vi "Object Tracking.vi"() -> ()   [LabVIEW 2019]
doc: "This example demonstrates the Traditional MeanShift algorithm to track an object in the image."
panel:
  in  "Stop":bool
  in  "Delay (s.)":dbl(slide) scale=0.0..2.0
  out "Image":T1(plugin-control)
  # "Overview: Demonstrate the Traditional MeanShift algorithm to track an object in the image.\nRequirements: LabVIEW Full Development System and Vision Development Module.\nInstructions: Run the VI."
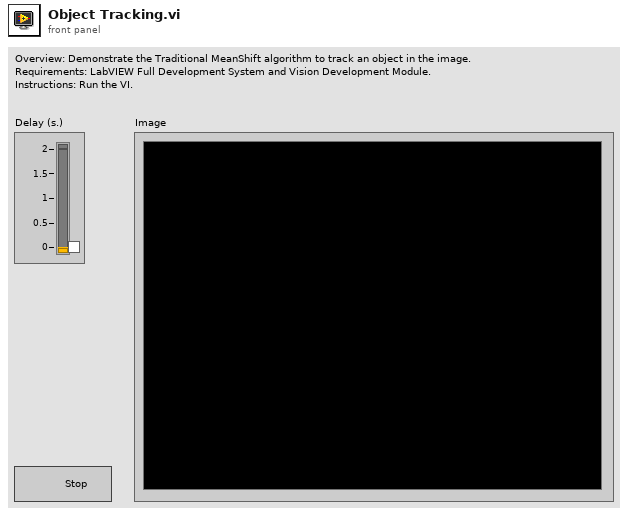
[diagram p1: front panel]
types:
  T1 = typedef "IMAQ Image.ctl" = refnum<image>
  T2 = cluster{"Number of Histogram Bins":i32, "Blending Parameter (%)":dbl, "Maximum Iterations":i32}
  T3 = typedef "Image Type" = u32
  T4 = typedef "IMAQ Object Tracking Session.ctl" = refnum<k20>
  T5 = typedef "IMAQ AVI2 Refnum.ctl" = refnum<k20>
  T6 = typedef "IMAQ Rectangle" = cluster{"Left":i32, "Top":i32, "Right":i32, "Bottom":i32, "Rotation":dbl}
  T7 = typedef "ROI Descriptor" = cluster{"Global Rectangle":i32[], "Contours":cluster{"ID":enum32{"External", "Internal"}, "Type":u32, "Coordinates":i32[]}[]}
  T8 = cluster{"Label":string, "Score":i32, "Angle":dbl, "Location":cluster{"X":dbl, "Y":dbl}, "Bounding Box":cluster{"X":dbl, "Y":dbl}[], "Object Found?":bool}[]
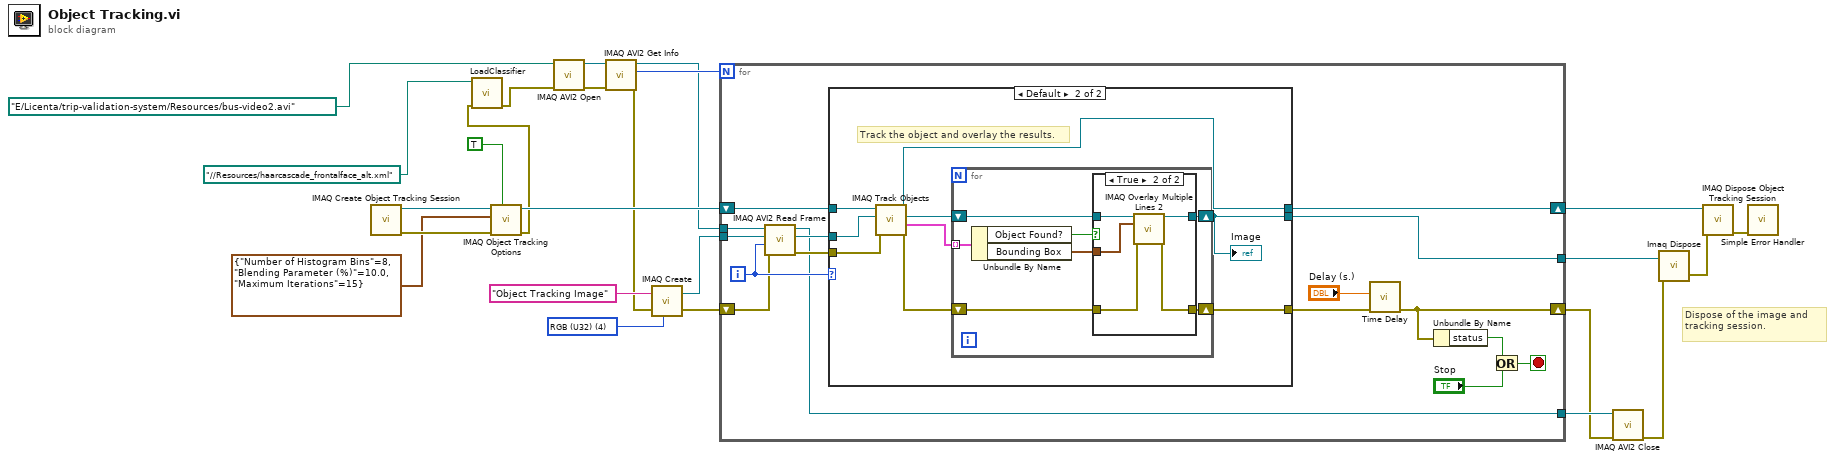
[diagram p0: block diagram]
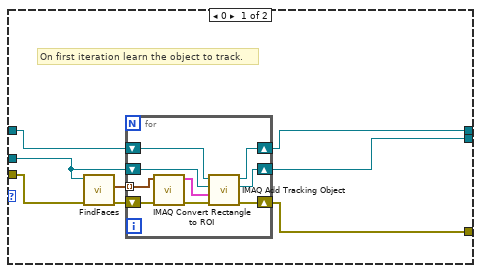
[diagram p2: hidden frame]
diagram:
  w12 = T3 4 items=["Grayscale (U8)", "Grayscale (I16)", "Grayscale (SGL)", "Complex (CSG)", "RGB (U32)", "HSL (U32)", "RGB (U64)", "Grayscale (U16)"] ("Image Type")
  # "Dispose of the image and tracking session."
  n1 = call "IMAQ Create Object Tracking Session"() -> ("error out"=w18:errorcluster, "Object Tracking Session"=w21:T4)  [unwired: 1 in, 9 out]
  n2 = call-poly "IMAQ Object Tracking Options"("Get/Set (Get)"=TRUE, "error in (no error)"=w18, "Mean Shift Options in"=T2 {"Number of Histogram Bins"=8, "Blending Parameter (%)"=10.0, "Maximum Iterations"=15}, "Object Tracking Session In"=w21) -> ("error out"=w4:errorcluster, "Object Tracking Session Out"=w20:T4)  [unwired: 5 in, 1 out]
  n3 = call "LoadClassifier.vi"("error in (no error)"=w4, "faceCascadePath"=path "../../Resources/haarcascade_frontalface_alt.xml" ("Face Cascade Path")) -> ("error out"=w3:errorcluster)  [unwired: 9 in]
  n4 = call "IMAQ AVI2 Open"("error in (no error)"=w3, "AVI File Path"=path "E:/Licenta/trip-validation-system/Resources/bus-video2.avi") -> ("error out"=w16:errorcluster, "AVI Refnum"=w17:T5)  [unwired: 8 in]
  n5 = call "IMAQ AVI2 Get Info"("error in (no error)"=w16, "AVI Refnum"=w17) -> ("error out"=w13:errorcluster, "Number of Frames"=w15:u32, "AVI Refnum (duplicate)"=w11:T5)  [unwired: 5 in, 2 out]
  n6 = call "IMAQ Create"("Image Name"="Object Tracking Image", "Image Type"=w12, "error in (no error)"=w13) -> ("New Image"=w10:T1, "error out"=w9:errorcluster)  [unwired: 2 in]
  n7 = for {
    N: w15 -> [_]
    tunnel: [w40] -> w25
    shift-right: [w38] -> w24
    shift-left: w20 -> [w39]
    tunnel: w11 -> [w35]
    tunnel: w10 -> [w34]
    shift-right: [w27] -> w7
    shift-left: w9 -> [w28]
    tunnel: [w26] -> w8
    i -> [w31]
    stop <- w29 stop-if-true
    n8 = call "IMAQ AVI2 Read Frame"("error in (no error)"=w28, "Frame Number"=w31, "Image"=w34, "AVI Refnum"=w35) -> ("error out"=w32:errorcluster, "Image Out"=w33:T1, "AVI Refnum (duplicate)"=w26:T5)  [unwired: 5 in]
    n9 = case shown="Default" w31 {
      tunnel: [w46 w67] -> w38
      tunnel: [w48 w65] -> w40
      tunnel: [w47 w62] -> w36
      tunnel: w39 -> [w49 w64]
      tunnel: w33 -> [w45 w61]
      tunnel: w32 -> [w44 w60]
      frame 0 {
        # "On first iteration learn the object to track."
        n10 = call "FindFaces.vi"("error in"=w44, "Image In"=w45) -> ("error out"=w43:errorcluster, "Faces"=w42:T6[])  [unwired: 7 in, 1 out]
        n11 = for {
          shift-right: [w55] -> w46
          shift-left: w49 -> [w58]
          shift-right: [w57] -> w48
          shift-left: w45 -> [w52]
          shift-right: [w56] -> w47
          shift-left: w43 -> [w51]
          tunnel: w42 -> [w50] mode=indexing
          n12 = call "IMAQ Convert Rectangle to ROI"("error in (no error)"=w51, "Rectangle"=w50) -> ("error out"=w54:errorcluster, "ROI Descriptor"=w53:T7)  [unwired: 7 in]
          n13 = call "IMAQ Add Tracking Object"("error in (no error)"=w54, "ROI Descriptor"=w53, "Image"=w52, "Object Tracking Session In"=w58) -> ("error out"=w56:errorcluster, "Image (duplicate)"=w57:T1, "Object Tracking Session Out"=w55:T4)  [unwired: 1 in, 4 out]
        }
      }
      frame Default {
        # "Track the object and overlay the results."
        n14 = call "IMAQ Track Objects"("error in (no error)"=w60, "Image"=w61, "Object Tracking Session In"=w64) -> ("error out"=w63:errorcluster, "Objects (pixel)"=w59:T8, "Image (duplicate)"=w66:T1, "Object Tracking Session Out"=w67:T4)  [unwired: 1 in, 4 out]
        n15 = for {
          shift-right: [w73] -> w65
          shift-left: w66 -> [w74]
          shift-right: [w70] -> w62
          shift-left: w63 -> [w71]
          tunnel: w59 -> [w68] mode=indexing
          n16 = Unbundle By Name(w68) -> ("Object Found?"=w69:bool, "Bounding Box"=w72:cluster{"X":dbl, "Y":dbl}[])
          n17 = case shown="True" w69 {
            tunnel: w74 -> [w75 w81]
            tunnel: [w75 w80] -> w73
            tunnel: w72 -> [_ w79]
            tunnel: w71 -> [w76 w78]
            tunnel: [w76 w77] -> w70
            frame False {
            }
            frame True {
              n18 = call "IMAQ Overlay Multiple Lines 2"("Image"=w81, "Line End Points"=w79, "error in (no error)"=w78) -> ("Image Out"=w80:T1, "error out"=w77:errorcluster)  [unwired: 5 in, 6 out]
            }
          }
        }
        "Image" <- w65
      }
    }
    n19 = call "Time Delay"("error in (no error)"=w36, "Delay Time (s)"="Delay (s.)") -> ("error out"=w27:errorcluster)  [unwired: 9 in]
    n20 = Unbundle By Name(w27) -> ("status"=w41:bool)
    n21 = Or(x=w41, y="Stop") -> (x .or. y?=w29:bool)
  }
  n22 = call "IMAQ AVI2 Close"("error in (no error)"=w7, "AVI Refnum"=w8) -> ("error out"=w6:errorcluster)  [unwired: 9 in]
  n23 = call "Imaq Dispose"("Image"=w25, "error in (no error)"=w6) -> ("error out"=w23:errorcluster)  [unwired: 1 in, 3 out]
  n24 = call "IMAQ Dispose Object Tracking Session"("error in (no error)"=w23, "Object Tracking Session"=w24) -> ("error out"=w22:errorcluster)  [unwired: 9 out]
  n25 = call <vilib>:"Simple Error Handler.vi"("error in (no error)"=w22) -> ()  [unwired: 1 in, 8 out]
